vi "Check_Database.vi"(2 "INFO":string="none", 3 "REQ":i32=1, 4 "STID":i32=1, 5 "RFID":string="39BC6D91") -> (0 "NAME":string, 1 "PERMISSION":string)   [LabVIEW 2014]
uses:
  <vilib>/httpClient/LabVIEWHTTPClient.lvlib
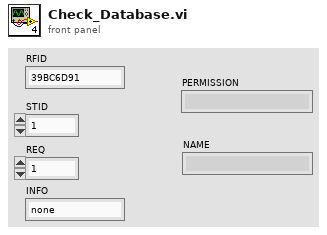
[diagram p1: front panel]
types:
  T1 = typedef "LabVIEWHTTPClient.lvlib/ClientHandle.ctl" = refnum<k1>
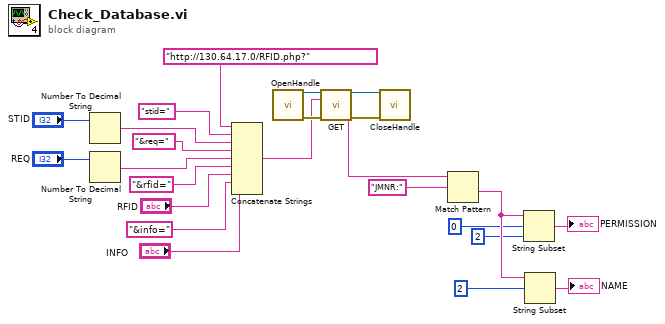
[diagram p0: block diagram]
diagram:
  n1 = Number To Decimal String(number="STID") -> (decimal integer string=w15:string)  [unwired: 1 in]
  n2 = Number To Decimal String(number="REQ") -> (decimal integer string=w1:string)  [unwired: 1 in]
  n3 = Concatenate Strings("http://130.64.17.0/RFID.php?" ("string"), "stid=" ("string"), w15, "&req=" ("string"), w1, "&rfid=" ("string"), "RFID", "&info=" ("string"), "INFO") -> (w19:string)
  n4 = call <vilib>:"OpenHandle.vi"() -> ("client handle out"=w23:T1, "error out"=w22:errorcluster)  [unwired: 14 in]
  n5 = call <vilib>:"GET.vi"("client handle"=w23, "url"=w19, "error in (no error)"=w22) -> ("client handle out"=w20:T1, "body"=w24:string, "error out"=w21:errorcluster)  [unwired: 9 in, 1 out]
  n6 = call <vilib>:"CloseHandle.vi"("client handle"=w20, "error in (no error)"=w21) -> ()  [unwired: 13 in, 1 out]
  n7 = Match Pattern(string=w24, regular expression="JMNR:") -> (after substring=w9:string)  [unwired: 1 in, 3 out]
  n8 = String Subset(string=w9, offset (0)=0, length (rest)=2 ("length (rest)")) -> (substring=→"PERMISSION":string)
  n9 = String Subset(string=w9, offset (0)=2) -> (substring=→"NAME":string)  [unwired: 1 in]
